vi "RTS Extract TCP Data Column.vi"(0 "Chamber 1 Socket":string[][](array[string]), 5 "Extract Column":i32=73, 11 "Error In":errorcluster) -> (2 "Station 1":i32, 3 "Station 2":i32, 4 "Station 3":i32, 6 "Station 4":i32, 8 "Station 5":i32, 10 "Station 6":i32, 13 "Station 8":i32, 14 "Station 7":i32, 15 "Error Out":errorcluster)   [LabVIEW 2016]
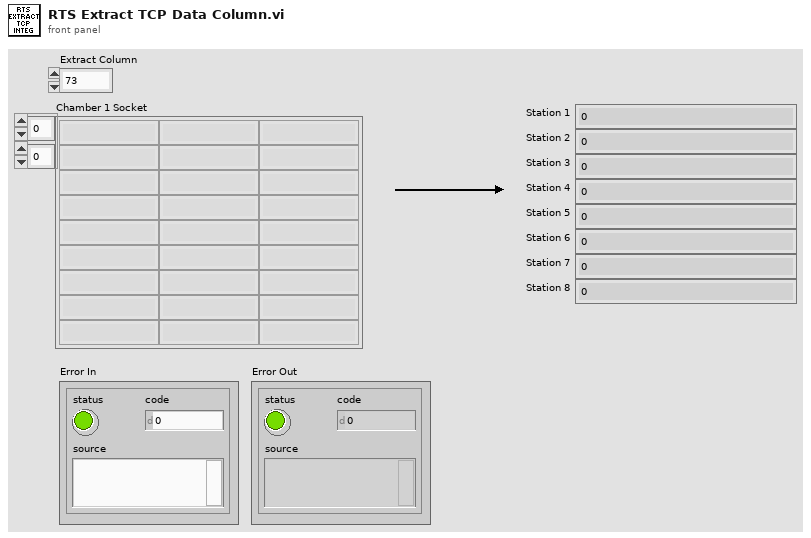
[diagram p1: front panel]
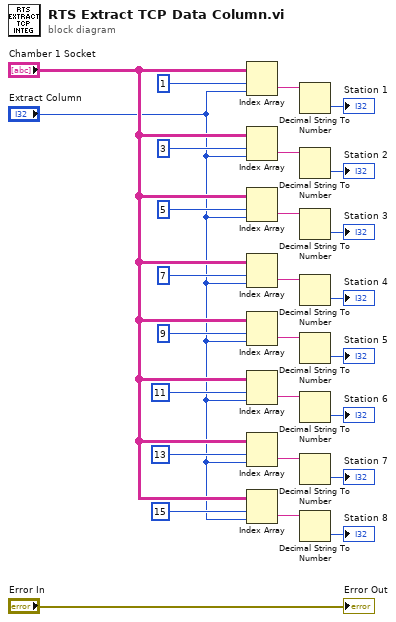
[diagram p0: block diagram]
diagram:
  n1 = Index Array(array="Chamber 1 Socket", index (row)=1, index (col)="Extract Column") -> (element=w18:string)
  n2 = Index Array(array="Chamber 1 Socket", index (row)=3, index (col)="Extract Column") -> (element=w17:string)
  n3 = Index Array(array="Chamber 1 Socket", index (row)=5, index (col)="Extract Column") -> (element=w16:string)
  n4 = Index Array(array="Chamber 1 Socket", index (row)=7, index (col)="Extract Column") -> (element=w15:string)
  n5 = Index Array(array="Chamber 1 Socket", index (row)=9, index (col)="Extract Column") -> (element=w14:string)
  n6 = Index Array(array="Chamber 1 Socket", index (row)=11, index (col)="Extract Column") -> (element=w13:string)
  n7 = Index Array(array="Chamber 1 Socket", index (row)=13, index (col)="Extract Column") -> (element=w12:string)
  n8 = Index Array(array="Chamber 1 Socket", index (row)=15, index (col)="Extract Column") -> (element=w11:string)
  n9 = Decimal String To Number(string=w18) -> (number=→"Station 1":i32)  [unwired: 2 in, 1 out]
  n10 = Decimal String To Number(string=w17) -> (number=→"Station 2":i32)  [unwired: 2 in, 1 out]
  n11 = Decimal String To Number(string=w16) -> (number=→"Station 3":i32)  [unwired: 2 in, 1 out]
  n12 = Decimal String To Number(string=w15) -> (number=→"Station 4":i32)  [unwired: 2 in, 1 out]
  n13 = Decimal String To Number(string=w14) -> (number=→"Station 5":i32)  [unwired: 2 in, 1 out]
  n14 = Decimal String To Number(string=w13) -> (number=→"Station 6":i32)  [unwired: 2 in, 1 out]
  n15 = Decimal String To Number(string=w12) -> (number=→"Station 7":i32)  [unwired: 2 in, 1 out]
  n16 = Decimal String To Number(string=w11) -> (number=→"Station 8":i32)  [unwired: 2 in, 1 out]
  "Error Out" <- "Error In"
